vi "Gather Subpanel References.vi"() -> (3 "subpanel array":refnum<vi>[](array[refnum]))   [LabVIEW 2020]
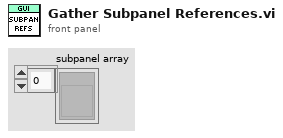
[diagram p1: front panel]
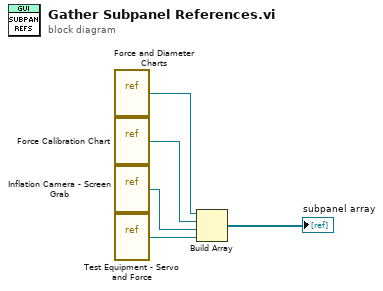
[diagram p0: block diagram]
diagram:
  n1 = vi-ref "Force and Diameter Charts.vi"() -> (w1:refnum<vi>)
  n2 = vi-ref "Force Calibration Chart.vi"() -> (w3:refnum<vi>)
  n3 = vi-ref "Inflation Camera - Screen Grab.vi"() -> (w4:refnum<vi>)
  n4 = vi-ref "Test Equipment - Servo and Force.vi"() -> (w2:refnum<vi>)
  n5 = Build Array(w1, w3, w4, w2) -> (→"subpanel array":refnum<vi>[])
